vi "Get All CD Item Property Values.vi"(8 "error in (no error)":errorcluster, 11 "CD Parameter Manager in":refnum<class "CD Parameter Manager.lvclass">) -> (0 "error out":errorcluster, 3 "CD Parameter Manager out":refnum<class "CD Parameter Manager.lvclass">)   [LabVIEW 2019, in "CD Parameter Manager API.lvlib" / "CD Parameter Manager.lvclass"]
uses:
  CD Parameter Manager.lvclass
  CD Parameter Manager.lvclass/CD Parameter Manager.ctl
  Parameter Class/Parameter.lvclass
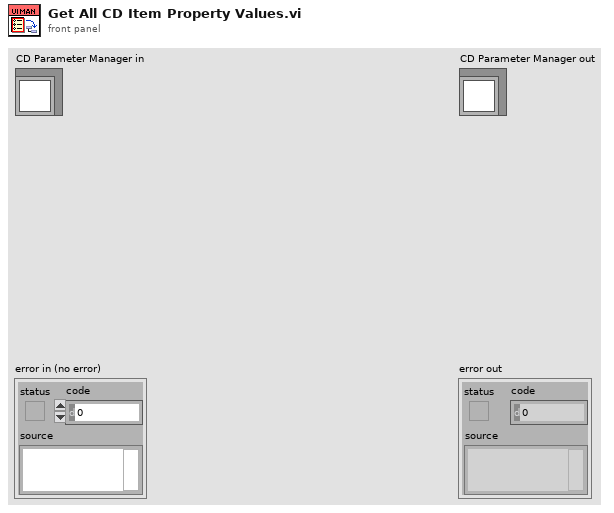
[diagram p1: front panel]
types:
  T1 = cluster{"Group name":string, "Controls":refnum<class "Parameter.lvclass">[]}[]
  T2 = typedef "Custom Device API.lvlib/Custom Device Item Ref.ctl" = u64
  T3 = cluster{"Group name":string, "Controls":refnum<class "Parameter.lvclass">[]}
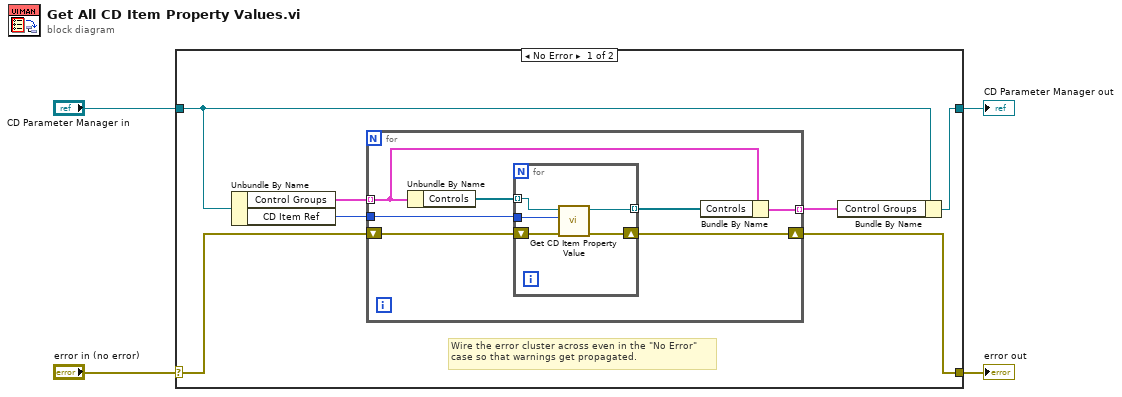
[diagram p0: block diagram]
diagram:
  n1 = case shown="No Error" "error in (no error)" {
    selector: "error in (no error)" -> [w10 w25]
    tunnel: [w6 w25] -> w3
    tunnel: [w7 w24] -> w1
    tunnel: "CD Parameter Manager in" -> [w8 w24]
    frame No Error {
      # "Wire the error cluster across even in the \"No Error\"\ncase so that warnings get propagated."
      n2 = Unbundle By Name(w8) -> ("Control Groups"=w11:T1, "CD Item Ref"=w9:T2)
      n3 = for {
        tunnel: w11 -> [w14] mode=indexing
        tunnel: w9 -> [w17]
        shift-right: [w16] -> w6
        shift-left: w10 -> [w18]
        tunnel: [w12] -> w5 mode=indexing
        n4 = Unbundle By Name(w14) -> ("Controls"=w15:refnum<class "Parameter.lvclass">[])
        n5 = for {
          tunnel: w17 -> [w22]
          shift-right: [w21] -> w16
          shift-left: w18 -> [w23]
          tunnel: [w20] -> w13 mode=indexing
          tunnel: w15 -> [w19] mode=indexing
          n6 = call-dynamic "Get CD Item Property Value.vi"("error in (no error)"=w23, "CD Item Ref in"=w22, "Parameter in"=w19) -> ("error out"=w21:errorcluster, "Parameter out"=w20:refnum<class "Parameter.lvclass">)  [unwired: 7 in]
        }
        n7 = Bundle By Name(cluster=w14, "Controls"=w13) -> (w12:T3)
      }
      n8 = Bundle By Name(cluster=w8, "Control Groups"=w5) -> (w7:refnum<class "CD Parameter Manager.lvclass">)
    }
    frame Error {
    }
  }
  "error out" <- w3
  "CD Parameter Manager out" <- w1
